vi "Test_NestedActorError_CollectSibling_RelayErrorToCaller.vi"(8 "error in (no error)":errorcluster, 11 "TestCase in":refnum<class "TestLaunchAndShutdown.lvclass">) -> (0 "error out":errorcluster, 3 "TestCase out":refnum<class "TestLaunchAndShutdown.lvclass">)   [LabVIEW 2020, in "TestLaunchAndShutdown.lvclass"]
uses:
  TestLaunchAndShutdown.lvclass
  TestLaunchAndShutdown.lvclass/TestLaunchAndShutdown.ctl
  24bf8875-c008-4f22-9bfa-88e42476d167.vi
  Source/IModel/IModel/IModel.lvclass
  <vilib>/ActorFramework/Actor/Actor.lvclass
  Source/Mediator/Mediator/Mediator.lvclass
  modules/composed-event-logger/Source/String Control Sink/String Control Sink.lvclass
  modules/composed-event-logger/Source/Composed Log/Types/Log Level.ctl
  modules/composed-event-logger/Source/Composed Log/Composed Log.lvlib
  modules/composed-event-logger/Source/String Formats/String Expression Format/String Expression Format.lvclass
  Doubles/ModelLaunchesActor/ModelLaunchesActor.lvclass
  Doubles/ActorGeneratesError/ActorGeneratesError.lvclass
  Doubles/RootModelNotifiesWhenStopped/RootModelNotifiesWhenStopped.lvclass
  C:/Git/mva-core/Source/RootModel/RootModel/RootModel.lvclass
  C:/Git/mva-core/Source/IModel/IModel/IModel.lvclass
  C:/Git/mva-core/Source/IObserver/IObserver/IObserver.lvclass
  C:/Program Files (x86)/National Instruments/LabVIEW 2020/vi.lib/ActorFramework/Actor/Actor.lvclass
  C:/Git/mva-core/Test/Doubles/RootModelNotifiesWhenStopped/RootModelNotifiesWhenStopped.lvclass
  C:/Git/mva-core/Test/Doubles/ActorGeneratesError/ActorGeneratesError.lvclass
  C:/Git/mva-core/modules/composed-event-logger/Source/IStringFormat/IStringFormat.lvclass
  C:/Git/mva-core/modules/composed-event-logger/Source/String Formats/String Expression Format/String Expression Format.lvclass
  C:/Git/mva-core/Test/Doubles/ModelLaunchesActor/ModelLaunchesActor.lvclass
panel:
  in  "Full Log":string
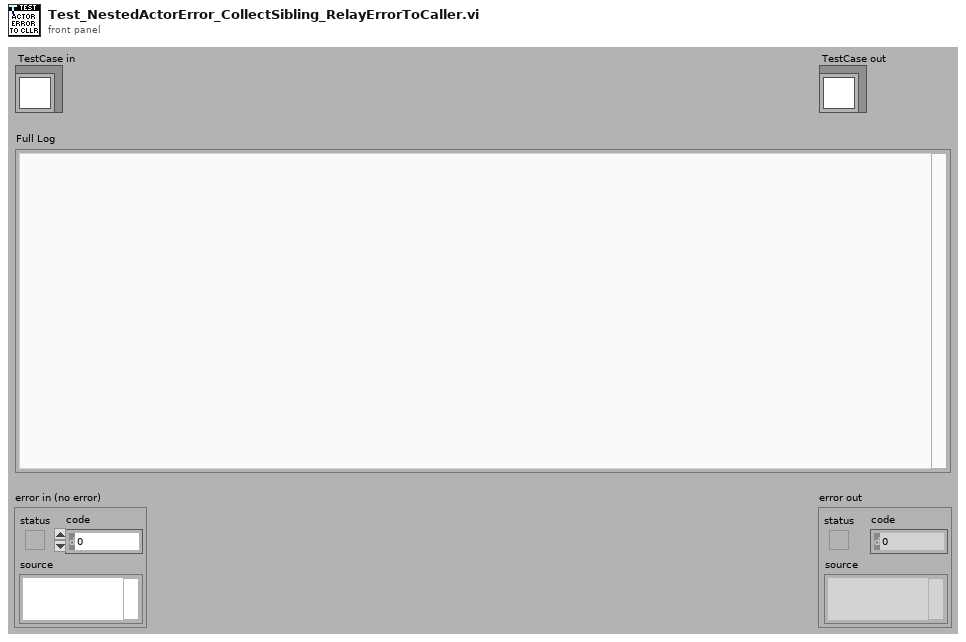
[diagram p1: front panel]
types:
  T1 = typedef "Composed Log.lvlib/Log Level.ctl" = enum16{"Debug", "Info", "Warning", "Error", "Critical"}
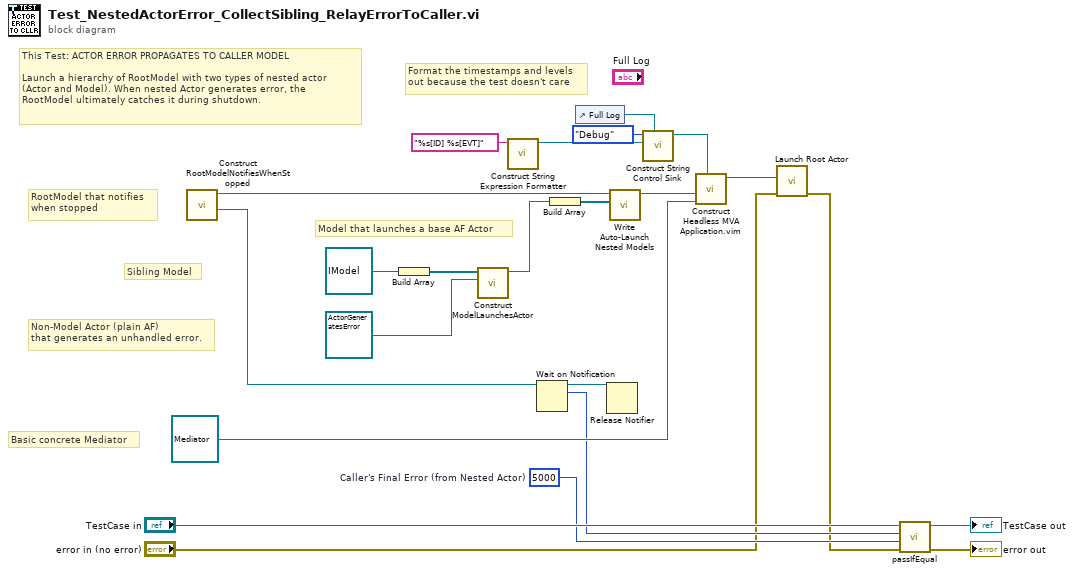
[diagram p0: block diagram]
diagram:
  w6 = 5000  # Caller's Final Error (from Nested Actor)
  # "Sibling Model"
  # "This Test: ACTOR ERROR PROPAGATES TO CALLER MODEL\n\nLaunch a hierarchy of RootModel with two types of nested actor\n(Actor and Model). When nested Actor generates error, the\nRootModel ultimately catches it during shutdown."
  # "Non-Model Actor (plain AF)\nthat generates an unhandled error."
  # "Model that launches a base AF Actor"
  # "Format the timestamps and levels\nout because the test doesn't care"
  # "RootModel that notifies\nwhen stopped"
  # "Basic concrete Mediator"
  n1 = call "Construct RootModelNotifiesWhenStopped.vi"() -> ("Final Error Notifier"=w1:refnum<notifier>, "RootModelNotifiesWhenStopped out"=w2:refnum<class "RootModelNotifiesWhenStopped.lvclass">)  [unwired: 10 in]
  n2 = Build Array(refnum<class "IModel.lvclass"> refnum ("IModel.lvlib:IModel.lvclass")) -> (w9:refnum<class "IModel.lvclass">[])
  n3 = call "Construct ModelLaunchesActor.vi"("Actor to Launch"=refnum<class "ActorGeneratesError.lvclass"> refnum ("ActorGeneratesError.lvclass"), "Auto-Launch Nested Models"=w9) -> ("ModelLaunchesActor out"=w10:refnum<class "ModelLaunchesActor.lvclass">)  [unwired: 9 in]
  n4 = call "Construct String Expression Formatter.vi"("Format Specifier"="%s[ID] %s[EVT]") -> ("String Expression Format out"=w13:refnum<class "String Expression Format.lvclass">)  [unwired: 9 in, 1 out]
  n5 = Wait on Notification(notifier=w1) -> (notifier out=w8:refnum<notifier>, notification=w7:i32)  [unwired: 3 in, 2 out]
  n6 = Build Array(w10) -> (w20:refnum<class "ModelLaunchesActor.lvclass">[])
  n7 = control-ref of="Full Log"() -> (w15:refnum<vi>)
  n8 = Release Notifier(notifier=w8) -> ()  [unwired: 2 in, 3 out]
  n9 = call "Write Auto-Launch Nested Models.vi"("Auto-Launch Nested Models"=w20, "IModel In"=w2) -> ("IModel Out"=w19:refnum<class "RootModelNotifiesWhenStopped.lvclass">)  [unwired: 9 in]
  n10 = call "Construct String Control Sink.vi"("Str Refnum"=w15, "LogFormat"=w13, "LogLevel"=Log_Level."Debug") -> ("String Control Sink out"=w16:refnum<class "String Control Sink.lvclass">)  [unwired: 8 in]
  n11 = call "Construct Headless MVA Application.vim"("Event Log Sink(s)"=w16, "Mediator Type"=refnum<class "Mediator.lvclass"> refnum ("Mediator.lvlib:Mediator.lvclass"), "RootModel in"=w19) -> ("RootModel out"=w18:refnum<class "RootModelNotifiesWhenStopped.lvclass">)  [unwired: 8 in]
  n12 = call <vilib>:"Launch Root Actor.vi"("error in (no error)"="error in (no error)", "Actor"=w18) -> ("error out"=w4:errorcluster)  [unwired: 8 in, 1 out]
  n13 = call-dynamic "passIfEqual.vi"("error in (no error)"=w4, "y"=w6, "x"=w7, "TestCase in"="TestCase in") -> ("error out"=→"error out":errorcluster, "TestCase out"=→"TestCase out":refnum<class "TestLaunchAndShutdown.lvclass">)  [unwired: 6 in]
